vi "VRES值.vi"(0 "XY":cluster{"数组":dbl[], "数组":dbl[]}[](array[cluster]), 1 "索引1":i32, 2 "索引2":i32) -> (15 "XY图 2":cluster{dbl[], dbl[]}[](graph))   [LabVIEW 2020]
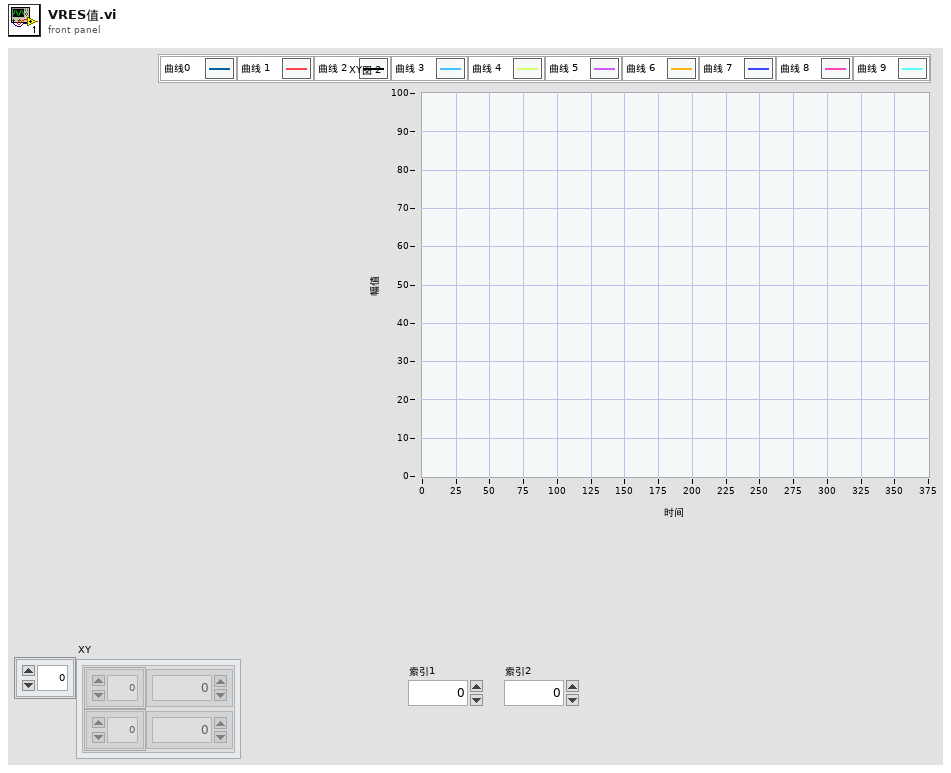
[diagram p1: front panel]
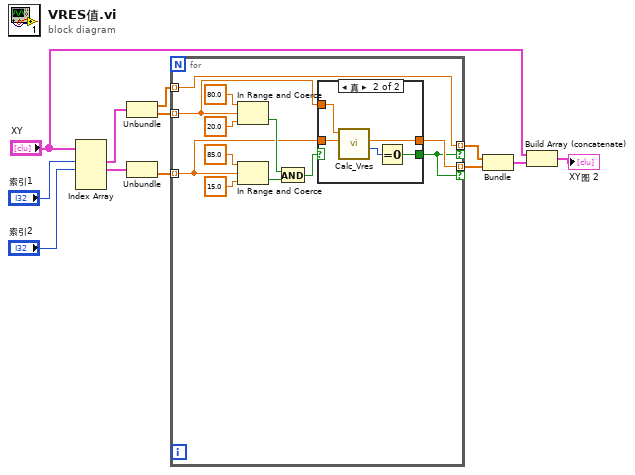
[diagram p0: block diagram]
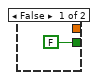
[diagram p2: hidden frame]
diagram:
  n1 = Index Array(array="XY", index #1="索引1", index #2="索引2") -> (element #1=w12:cluster{"数组":dbl[], "数组":dbl[]}, element #2=w11:cluster{"数组":dbl[], "数组":dbl[]})  [unwired: 2 in, 2 out]
  n2 = Unbundle(w12) -> ("数组"=w6:dbl[], "数组"=w10:dbl[])
  n3 = Unbundle(w11) -> ("数组"=w9:dbl[])  [unwired: 1 out]
  n4 = for {
    tunnel: w10 -> [w23] mode=indexing
    tunnel: w9 -> [w17] mode=indexing
    tunnel: [w24] -> w1 mode=indexing if=w18
    tunnel: w6 -> [w19] mode=indexing
    tunnel: [w19] -> w5 mode=indexing if=w18
    n5 = In Range and Coerce(upper limit=80.0 ("上限"), x=w23, lower limit=20.0 ("下限")) -> (In Range?=w20:bool)  [unwired: 1 out]
    n6 = In Range and Coerce(upper limit=85.0 ("上限"), x=w17, lower limit=15.0 ("下限")) -> (In Range?=w13:bool)  [unwired: 1 out]
    n7 = And(x=w20, y=w13) -> (x .and. y?=w14:bool)
    n8 = case shown="真" w14 {
      tunnel: [_ w30] -> w24
      tunnel: w17 -> [_ w29]
      tunnel: w23 -> [_ w28]
      tunnel: [FALSE w27] -> w18
      frame False {
      }
      frame True {
        n9 = call "Calc_Vres.vi"("S_Data in"=w29, "P_Data in"=w28) -> ("Vres_FD"=w26:i32, "Vres"=w30:dbl)  [unwired: 7 in, 1 out]
        n10 = Equal To 0?(x=w26) -> (x = 0?=w27:bool)
      }
    }
  }
  n11 = Bundle(w5, w1) -> (w8:cluster{dbl[], dbl[]})  [unwired: 1 in]
  n12 = Build Array (concatenate)("XY", w8) -> (→"XY图 2":cluster{"数组":dbl[], "数组":dbl[]}[])
